vi "parse_Inertia.vi"(4 "error in":errorcluster, 7 "msg in":string) -> (0 "error out":errorcluster, 2 "Inertia":T1, 3 "msg out":string)   [LabVIEW 2012]
doc: "Parses a message into an inertia"
uses:
  <userlib>/ROS for LabVIEW Software/ROS/MessageParsing/std_msgs/subs/parse_float64_scalar.vi
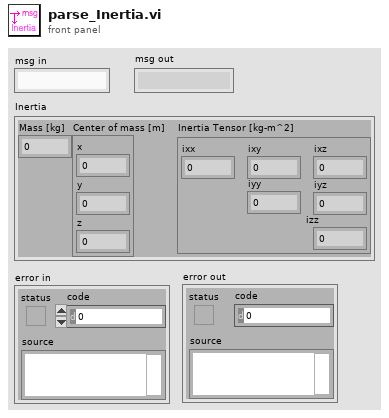
[diagram p1: front panel]
types:
  T1 = cluster{"Mass [kg]":dbl, "Center of mass [m]":cluster{"x":dbl, "y":dbl, "z":dbl}, "Inertia Tensor [kg-m^2]":cluster{"ixx":dbl, "ixy":dbl, "ixz":dbl, "iyy":dbl, "iyz":dbl, "izz":dbl}}
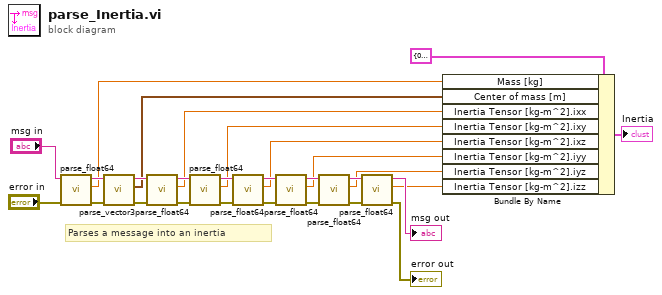
[diagram p0: block diagram]
diagram:
  # "Parses a message into an inertia"
  n1 = call-poly <userlib>:"parse_float64.vi"("error in"="error in", "msg in"="msg in") -> ("error out"=w18:errorcluster, "number"=w8:dbl, "msg out"=w27:string)  [unwired: 3 in]
  n2 = call <userlib>:"parse_vector3.vi"("error in"=w18, "msg in"=w27) -> ("error out"=w17:errorcluster, "Vector3"=w7:cluster{"x":dbl, "y":dbl, "z":dbl}, "msg out"=w26:string)  [unwired: 3 in]
  n3 = call-poly <userlib>:"parse_float64.vi"("error in"=w17, "msg in"=w26) -> ("error out"=w16:errorcluster, "number"=w6:dbl, "msg out"=w25:string)  [unwired: 3 in]
  n4 = call-poly <userlib>:"parse_float64.vi"("error in"=w16, "msg in"=w25) -> ("error out"=w15:errorcluster, "number"=w5:dbl, "msg out"=w24:string)  [unwired: 3 in]
  n5 = call-poly <userlib>:"parse_float64.vi"("error in"=w15, "msg in"=w24) -> ("error out"=w14:errorcluster, "number"=w4:dbl, "msg out"=w23:string)  [unwired: 3 in]
  n6 = call-poly <userlib>:"parse_float64.vi"("error in"=w14, "msg in"=w23) -> ("error out"=w13:errorcluster, "number"=w3:dbl, "msg out"=w22:string)  [unwired: 3 in]
  n7 = call-poly <userlib>:"parse_float64.vi"("error in"=w13, "msg in"=w22) -> ("error out"=w12:errorcluster, "number"=w2:dbl, "msg out"=w21:string)  [unwired: 3 in]
  n8 = call-poly <userlib>:"parse_float64.vi"("error in"=w12, "msg in"=w21) -> ("error out"=→"error out":errorcluster, "number"=w1:dbl, "msg out"=→"msg out":string)  [unwired: 3 in]
  n9 = Bundle By Name(cluster=T1 {"Mass [kg]"=0.0, "Center of mass [m]"={"x"=0.0, "y"=0.0, "z"=0.0}, "Inertia Tensor [kg-m^2]"={"ixx"=0.0, "ixy"=0.0, "ixz"=0.0, "iyy"=0.0, "iyz"=0.0, "izz"=0.0}} ("Inertia"), "Mass [kg]"=w8, "Center of mass [m]"=w7, "Inertia Tensor [kg-m^2].ixx"=w6, "Inertia Tensor [kg-m^2].ixy"=w5, "Inertia Tensor [kg-m^2].ixz"=w4, "Inertia Tensor [kg-m^2].iyy"=w3, "Inertia Tensor [kg-m^2].iyz"=w2, "Inertia Tensor [kg-m^2].izz"=w1) -> (→"Inertia":T1)
